vi "Trajectory Builder.vi"() -> ()   [LabVIEW 2018]
uses:
  2019 robot/Support Code/Availible Command systems for auto.ctl
  <vilib>/event_ctls.llb/lveventtype.ctl
panel:
  out "folder names":cluster{"name":string, "name":string}
  in  "Directory":bool
  in  "Tab Control":T1(tab)
  out "Duration (s)":dbl format="%#.4g"
  out "Distance (ft)":dbl format="%#.1g"
  out "WayPoints":cluster{"x":dbl, "y":dbl, "th":dbl}[](array[cluster]) {"th" format="%#_4g"}
  in  "Center Flip":bool
  in  "Snap to foot":bool
  in  "Angle Limiter":enum16{"90", "45", "15", "1"}(ring)=enum."15"
  in  "Snap robot to baseline":bool
  in  "Angular Accelerations":T2 {"Angular \nAccelerations" step=5.0}
  in  "Limits":T3={"Velocity (fps)"=6.0, "Accel (fps^2)"=15.0, "Jerk (fps^3)"=15.0} {"Jerk (fps^3)" min=0.0 step=1.0; "Accel (fps^2)" min=0.0; "Velocity (fps)" min=0.0}
  in  "Conditions":T4 {"vFinal (fps)" min=0.0; "vInitial (fps)" min=0.0}
  in  "Sample Period (s)":dbl=0.02
  in  "Unjank":bool
  in  "Turn \nAcceleration":bool=TRUE
  in  "Turn \nDeceleration":bool=TRUE
  out "Command Info":string
  in  "Reorder":bool
  in  "Commands":T5(array[cluster]) {"System" items=["Elevator", "Carriage Intake STOP", "Carriage Intake RUN"]}
  in  "Time (s)":dbl(slide) scale=-1.0..5.140000000000001 scale format="%#.1g"
  in  "Play":bool
  in  "Sub Dir 2":u16(ring)
  in  "Sub Dir 1":u16(ring) items=["Experimental", "Left", "Other", "Right"]
  out "fps":dbl[](graph)
  in  "Append":bool
  in  "Open":i32(listbox)
  in  "Filename":string
  in  "Save":bool
  in  "New":bool
  out "Picture":picture
  # "Directions:\nUse mouse to ...\n    move robot position (rectangle with arrow)\n    rotate robot (red arrow)\n    move waypoints (numbered circles)\nClick in open space to add a waypoint\nShift click to delete a waypoint\nHover over a waypoint and use arrow keys to nudge\n\nTime slider and Play button will run robot along path\nto test for collisions\n\nDirection and Destionation are folder selectors for files\n\nNew creates a new path at default location\n\nAppend creates a path"
  # "Nicotine"
  # "(20ms)"
  # "Interaction Options"
  # "Path Info"
  # "1"
  # "2"
  # "3"
  # "4"
  # "5"
  # "6"
  # "7"
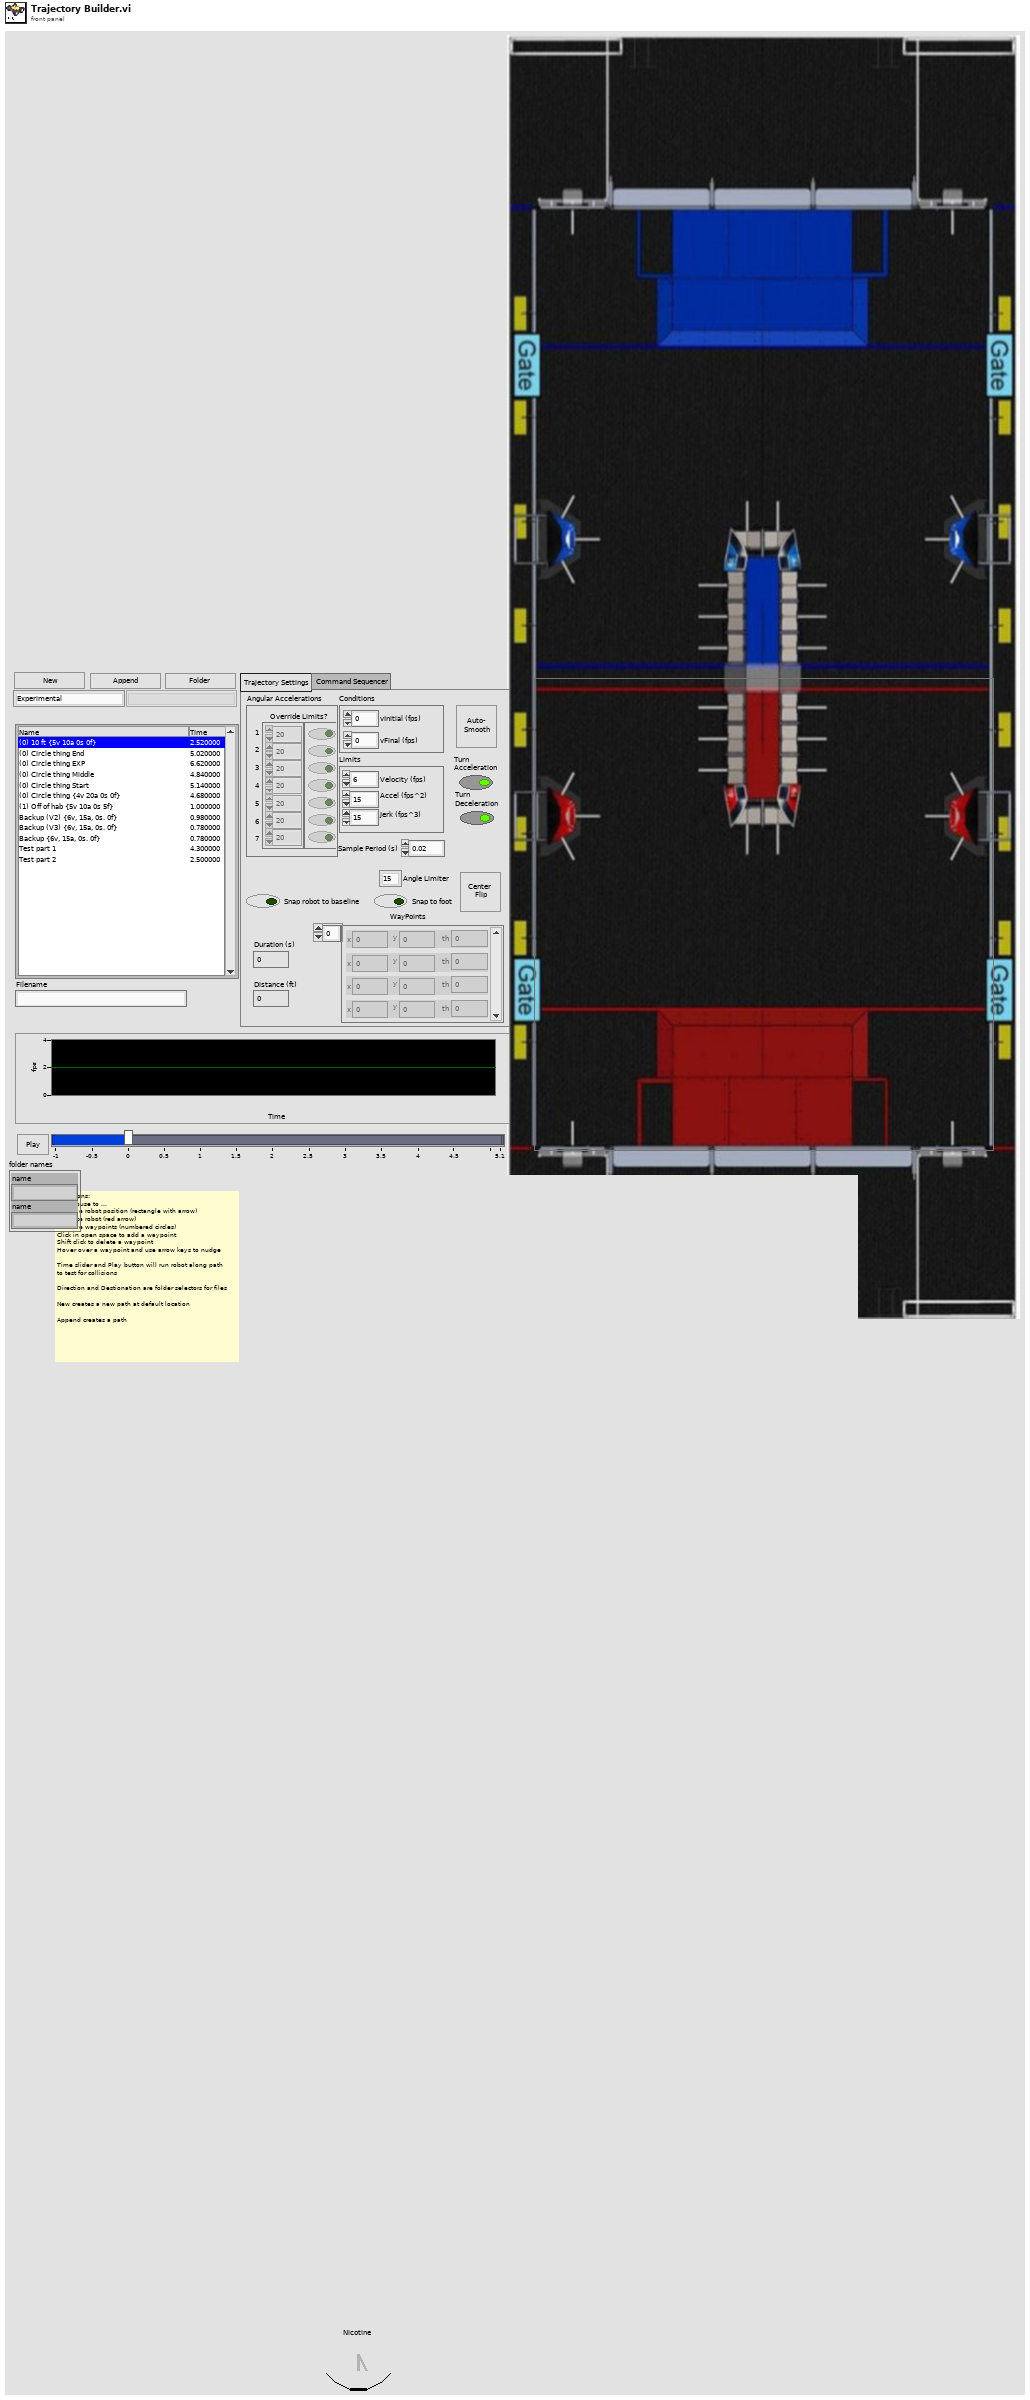
[diagram p1: front panel]
types:
  T1 = enum32{"Trajectory Settings", "Command Sequencer"}
  T2 = cluster{"Angular \nAccelerations":dbl[], "Override Limits?":bool[]}
  T3 = cluster{"Velocity (fps)":dbl, "Accel (fps^2)":dbl, "Jerk (fps^3)":dbl}
  T4 = cluster{"vInitial (fps)":dbl, "vFinal (fps)":dbl}
  T5 = cluster{"Time into Path":dbl, "System":u16, "Item Selected?":bool, "System Selection":u16}[]
  T6 = cluster{"Sample Period (s)":dbl, "Limits":cluster{"Velocity (fps)":dbl, "Acceleration (fps^2)":dbl, "Jerk (fps^3)":dbl}, "Conditions":cluster{"vInitial (fps)":dbl, "vFinal (fps)":dbl}, "output cluster":cluster{"Angular \nAccelerations":dbl[], "Override Limits?":bool[]}}
  T7 = cluster{"Segment Name":string, "Type":enum16{"Accel Straight", "Const Straight", "Blend", "Circle"}, "Traj Pos Points":cluster{"x":dbl, "y":dbl, "th":dbl}[], "Traj Vel Points":cluster{"V":dbl, "th":dbl}[], "Accel Index":i32, "Decel Index":i32}[]
  T8 = cluster{"Index":i32, "Pt Test Results":enum16{"Miss", "Rect Hit", "Arrow Hit"}}
  T9 = cluster{"Drag Object":cluster{"Index":i32, "x":dbl, "y":dbl}, "Hover Object":cluster{"Index":i32, "Pt Test Results":enum16{"Miss", "Rect Hit", "Arrow Hit"}}}
  T10 = cluster{"Trajectory Data":cluster{"Segment Name":string, "Type":enum16{"Accel Straight", "Const Straight", "Blend", "Circle"}, "Traj Pos Points":cluster{"x":dbl, "y":dbl, "th":dbl}[], "Traj Vel Points":cluster{"V":dbl, "th":dbl}[], "Accel Index":i32, "Decel Index":i32}[], "Points":cluster{"x":dbl, "y":dbl, "th":dbl}[], "Cluster":cluster{"Sample Period (s)":dbl, "Limits":cluster{"Velocity (fps)":dbl, "Acceleration (fps^2)":dbl, "Jerk (fps^3)":dbl}, "Conditions":cluster{"vInitial (fps)":dbl, "vFinal (fps)":dbl}, "output cluster":cluster{"Angular \nAccelerations":dbl[], "Override Limits?":bool[]}}}
  T11 = cluster{"Velocity":dbl, "Sample Time":dbl, "Accel":dbl}
  T12 = cluster{"Sample Period (s)":dbl, "Limits":cluster{"Velocity (fps)":dbl, "Acceleration (fps^2)":dbl, "Jerk (fps^3)":dbl}, "Conditions":cluster{"vInitial (fps)":dbl, "vFinal (fps)":dbl}}
  T13 = cluster{"Sample Period (s)":dbl, "Limits":cluster{"Velocity (fps)":dbl, "Acceleration (fps^2)":dbl, "Jerk (fps^3)":dbl}, "Conditions":cluster{"vInitial (fps)":dbl, "vFinal (fps)":dbl}, "Min Rads":dbl[]}
  T14 = typedef "Availible Command systems for auto.ctl" = u16
  T15 = cluster{"Time into Path":dbl, "System":T14, "Item Selected?":bool, "System Selection":T14}[]
  T16 = typedef "lveventtype.ctl" = enum32{"Null", "Timeout", "Annotation Menu Selection", "Annotation Menu Selection?", "App Instance Close", "App Instance Close?", "Autoscale Range Change", "Bookmark Info Change", "Cell Edit", "Cell Edit?", "Cursor Grab", "Cursor Grab?", "Cursor Menu Selection", "Cursor Menu Selection?", "Cursor Move", "Cursor Release", "Data Change", "Direction Change", "Display State Change", "Drag Ended", "Drag Enter", "Drag Leave", "Drag Over", "Drag Source Update", "Drag Starting", "Drag Starting?", "Drop", "Exec State Change", "Key Down", "Key Down?", "Key Repeat", "Key Repeat?", "Key Up", "Listbox Double Click", "Menu Activation?", "Menu Selection (App)", "Menu Selection? (App)", "Menu Selection (User)", "Mouse Down", "Mouse Down?", "Mouse Enter", "Mouse Leave", "Mouse Move", "Mouse Up", "Mouse Wheel", "NI Security User Change (App)", "Pane Size", "Panel Close", "Panel Close?", "Panel Resize", "Plot Attribute Change", "Scale Range Change", "Shortcut Menu Activation?", "Shortcut Menu Selection (App)", "Shortcut Menu Selection? (App)", "Shortcut Menu Selection (User)", "Tree Double Click", "Tree Drag", "Tree Drag?", "Tree Drop", "Tree Drop?", "Tree Item Close", "Tree Item Close?", "Tree Item Open", "Tree Item Open?", "User Event", "Value Change"}
  T17 = cluster{"Sample Period (s)":dbl, "Limits":cluster{"Velocity (fps)":dbl, "Accel (fps^2)":dbl, "Jerk (fps^3)":dbl}, "Conditions":cluster{"vInitial (fps)":dbl, "vFinal (fps)":dbl}, "Angular Accelerations":cluster{"Angular \nAccelerations":dbl[], "Override Limits?":bool[]}}
  T18 = typedef "LVPoint32TypeDef.ctl" = cluster{"Horizontal":i32, "Vertical":i32}
  T19 = cluster{"Shift":bool, "Ctrl":bool, "Alt":bool, "Cmd":bool, "Opt":bool}
  T20 = typedef "LVPositionTypeDef.ctl" = cluster{"Left":i32, "Top":i32}
  T21 = typedef "LVBoundsTypeDef.ctl" = cluster{"Width":u32, "Height":u32}
  T22 = cluster{"Velocity":dbl, "Accel":dbl, "Accel":dbl}
  T23 = cluster{"Velocity (fps)":dbl, "Acceleration (fps^2)":dbl, "Jerk (fps^3)":dbl}
  T24 = cluster{"Trajectory Data":cluster{"Segment Name":string, "Type":enum16{"Accel Straight", "Const Straight", "Blend", "Circle"}, "Traj Pos Points":cluster{"x":dbl, "y":dbl, "th":dbl}[], "Traj Vel Points":cluster{"V":dbl, "th":dbl}[], "Accel Index":i32, "Decel Index":i32}[], "Points":cluster{"x":dbl, "y":dbl, "th":dbl}[], cluster{"Sample Period (s)":dbl, "Limits":cluster{"Velocity (fps)":dbl, "Accel (fps^2)":dbl, "Jerk (fps^3)":dbl}, "Conditions":cluster{"vInitial (fps)":dbl, "vFinal (fps)":dbl}, "Angular Accelerations":cluster{"Angular \nAccelerations":dbl[], "Override Limits?":bool[]}}}
  T25 = cluster{"Snap robot to baseline":bool, "Snap to foot":bool, "Angle Limiter":enum16{"90", "45", "15", "1"}}
  T26 = cluster{i32, "Pt Test Results":enum16{"Miss", "Rect Hit", "Arrow Hit"}}
  T27 = cluster{"Drag Object":cluster{"Index":i32, "x":dbl, "y":dbl}, "Results":cluster{"Index":i32, "Pt Test Results":enum16{"Miss", "Rect Hit", "Arrow Hit"}}}
  T28 = cluster{"Trajectory Data":cluster{"Segment Name":string, "Type":enum16{"Accel Straight", "Const Straight", "Blend", "Circle"}, "Traj Pos Points":cluster{"x":dbl, "y":dbl, "th":dbl}[], "Traj Vel Points":cluster{"V":dbl, "th":dbl}[], "Accel Index":i32, "Decel Index":i32}[], "Updated Waypoints":cluster{"x":dbl, "y":dbl, "th":dbl}[], "Cluster":cluster{"Sample Period (s)":dbl, "Limits":cluster{"Velocity (fps)":dbl, "Accel (fps^2)":dbl, "Jerk (fps^3)":dbl}, "Conditions":cluster{"vInitial (fps)":dbl, "vFinal (fps)":dbl}, "Angular Accelerations":cluster{"Angular \nAccelerations":dbl[], "Override Limits?":bool[]}}}
  T29 = typedef "eventvkey.ctl" = enum16{"ASCII", "Enter", "Return", "Shift", "Ctrl", "Alt", "Cmd", "Opt", "Caps", "NumLock", "Clear", "Break", "Up", "Down", "Left", "Right", "Insert", "Delete", "Home", "End", "PageUp", "PageDown", "Escape", "Help", "Pause", "ScrollLock", "F1", "F2", "F3", "F4", "F5", "F6", "F7", "F8", "F9", "F10", "F11", "F12", "F13", "F14", "F15", "F16", "F17", "F18", "F19", "F20", "F21", "F22", "F23", "F24", "Play", "VolumeUp", "VolumeDown", "Mute", "Two Byte Char"}
  T30 = cluster{"Trajectory Data":cluster{"Segment Name":string, "Type":enum16{"Accel Straight", "Const Straight", "Blend", "Circle"}, "Traj Pos Points":cluster{"x":dbl, "y":dbl, "th":dbl}[], "Traj Vel Points":cluster{"V":dbl, "th":dbl}[], "Accel Index":i32, "Decel Index":i32}[], "Updated Waypoints":cluster{"x":dbl, "y":dbl, "th":dbl}[], cluster{"Sample Period (s)":dbl, "Limits":cluster{"Velocity (fps)":dbl, "Accel (fps^2)":dbl, "Jerk (fps^3)":dbl}, "Conditions":cluster{"vInitial (fps)":dbl, "vFinal (fps)":dbl}, "Angular Accelerations":cluster{"Angular \nAccelerations":dbl[], "Override Limits?":bool[]}}}
  T31 = cluster{"Horizontal":dbl, "Vertical":dbl, "th":dbl}
  T32 = cluster{"Name":string, "Color":u32, "Style":i32, "Point Style":i32, "Name Visible":bool, "Allow Drag":bool, "Annotation Mode":i32, "Plot":i32, "Index":i32, "Position":cluster{"X":dbl, "Y":dbl}, "X Scale":i32, "Y Scale":u32, "Show Arrow":bool, "Lock Name":bool, "Plot Area":i32, "Label Offset":cluster{"X":dbl, "Y":dbl}}[]
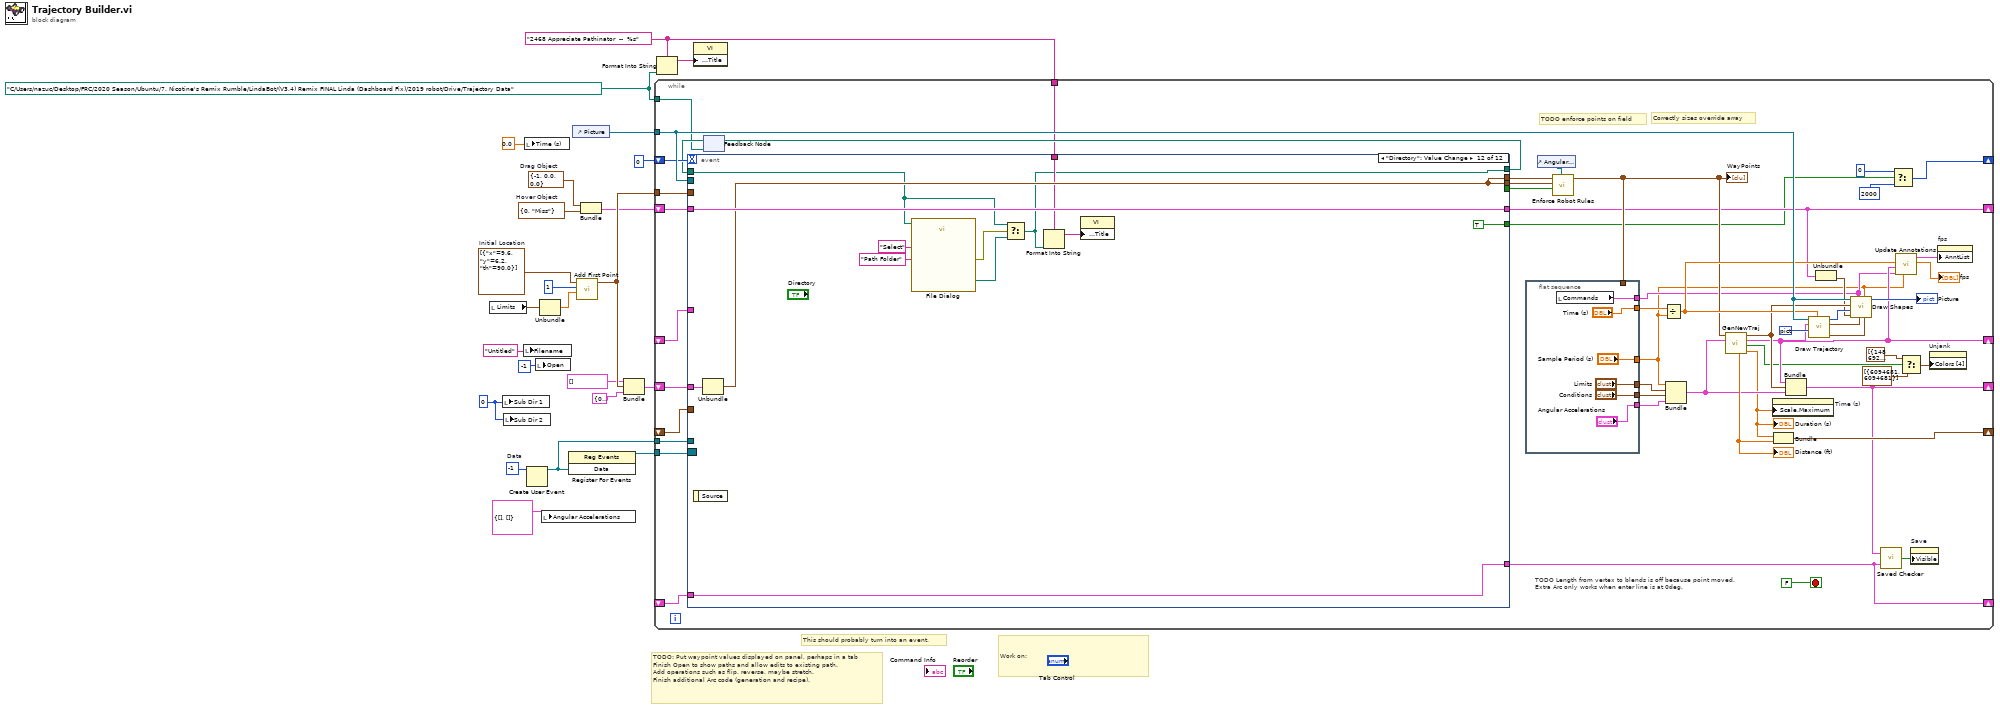
[diagram p0: block diagram]
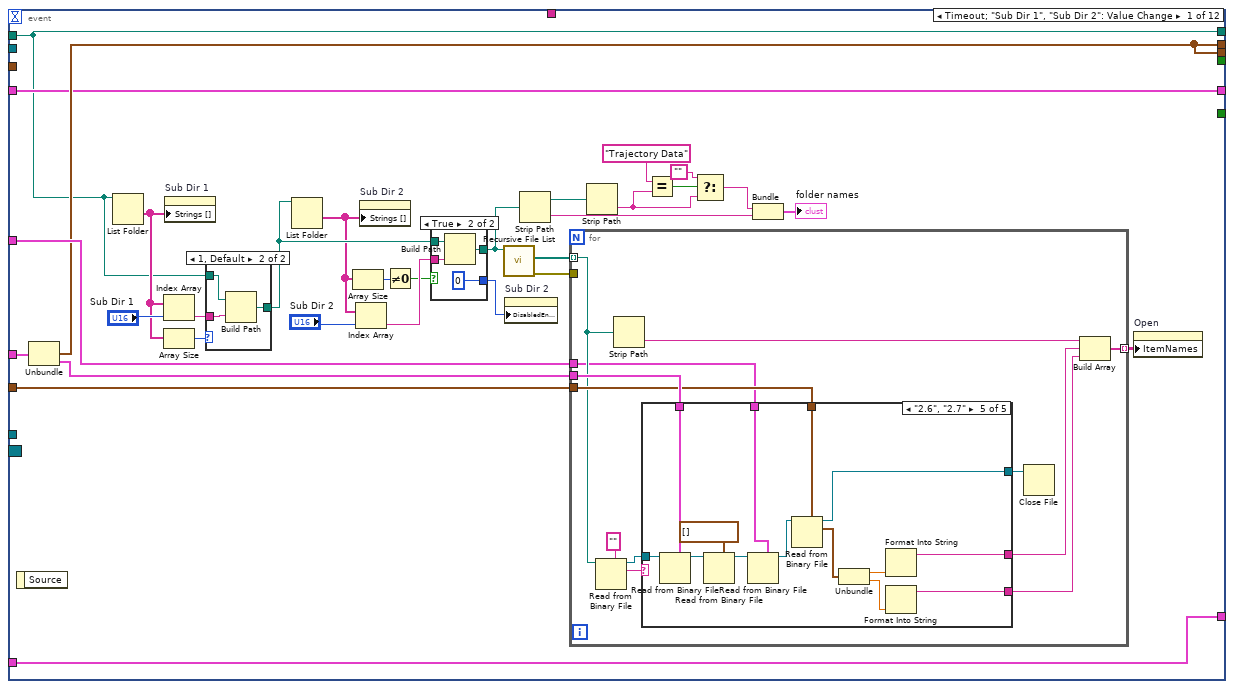
[diagram p2: hidden frame]
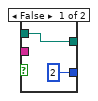
[diagram p4: hidden frame]
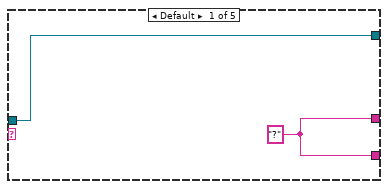
[diagram p5: hidden frame]
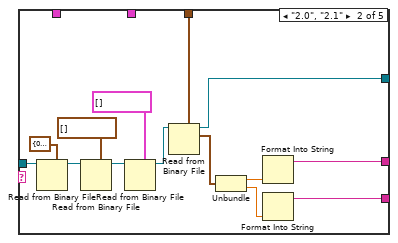
[diagram p6: hidden frame]
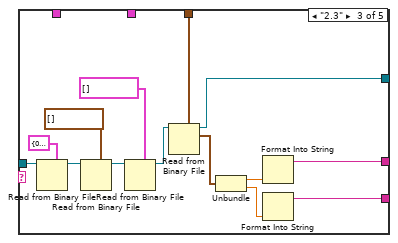
[diagram p7: hidden frame]
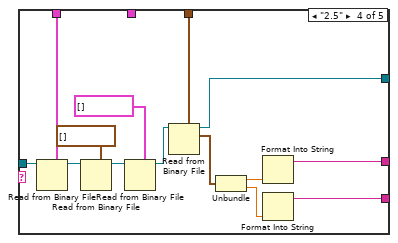
[diagram p8: hidden frame]
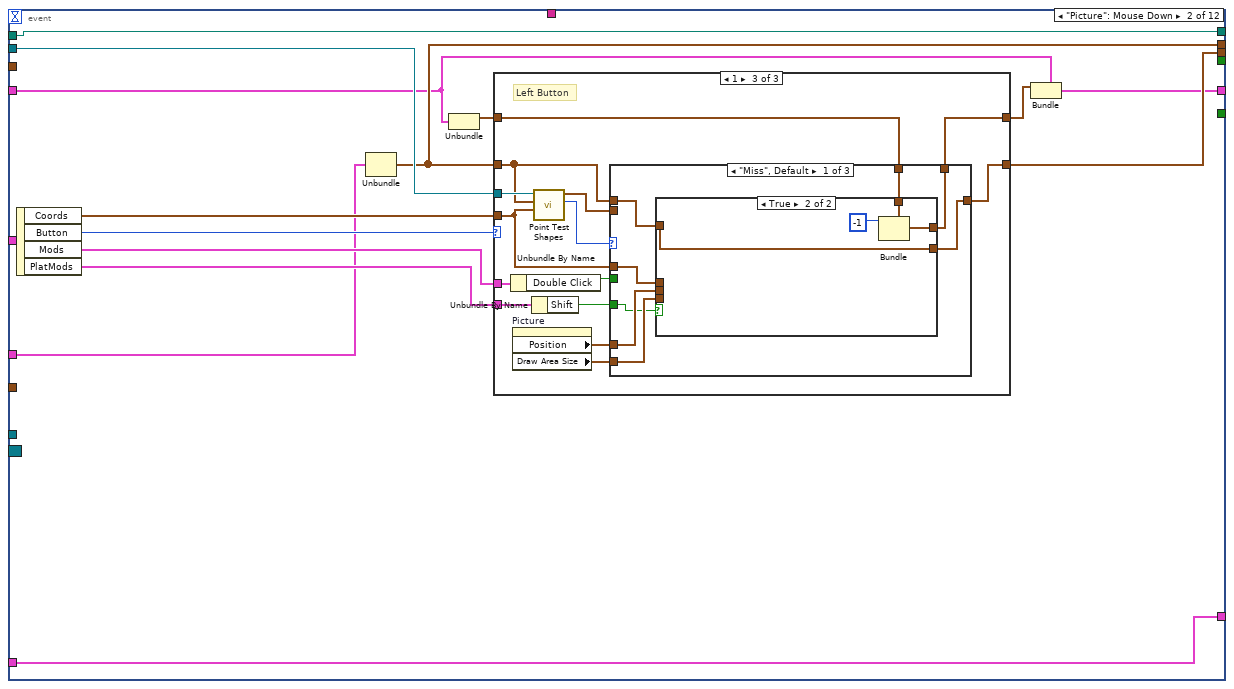
[diagram p9: hidden frame]
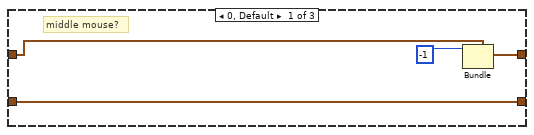
[diagram p10: hidden frame]
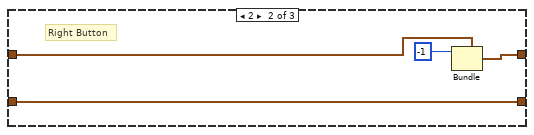
[diagram p11: hidden frame]
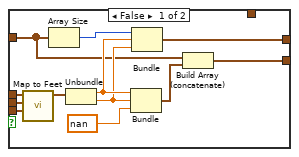
[diagram p12: hidden frame]
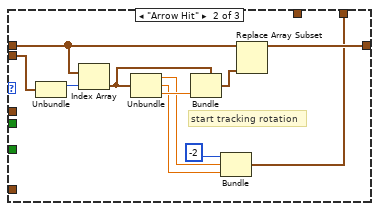
[diagram p13: hidden frame]
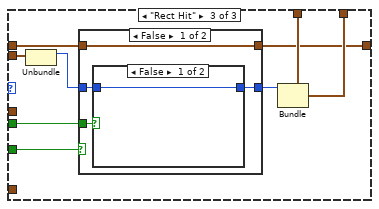
[diagram p14: hidden frame]
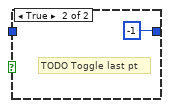
[diagram p15: hidden frame]
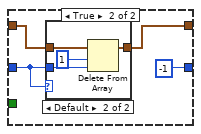
[diagram p16: hidden frame]
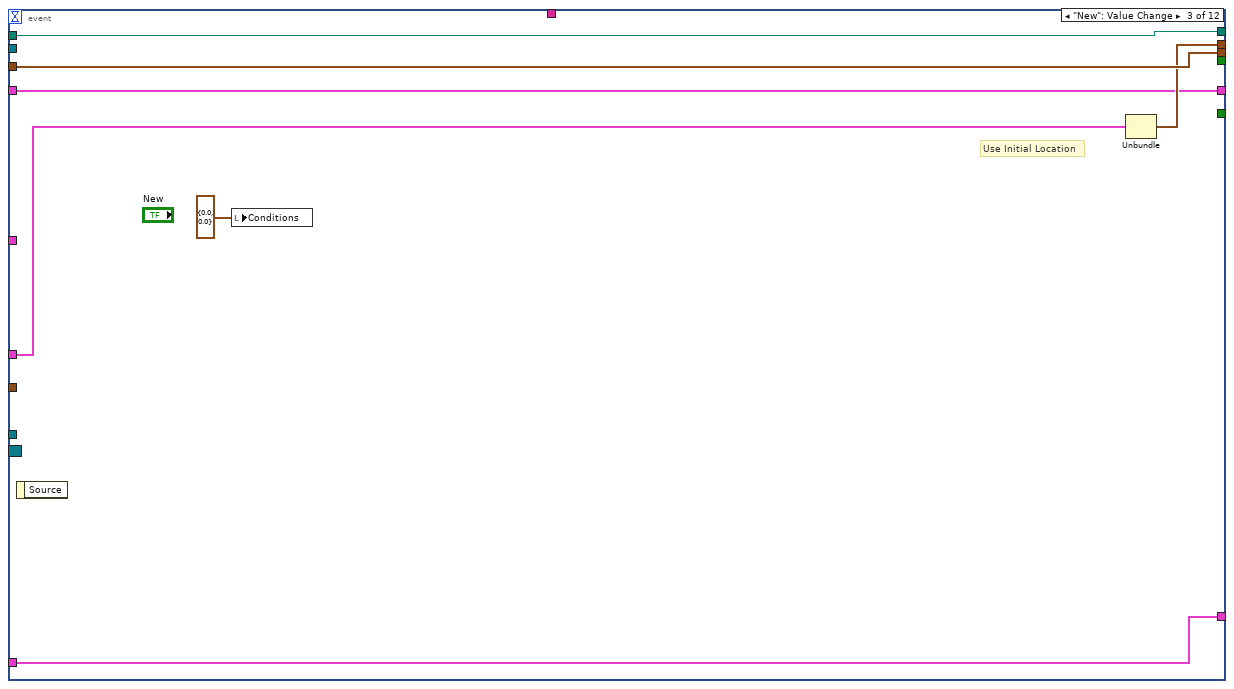
[diagram p18: hidden frame]
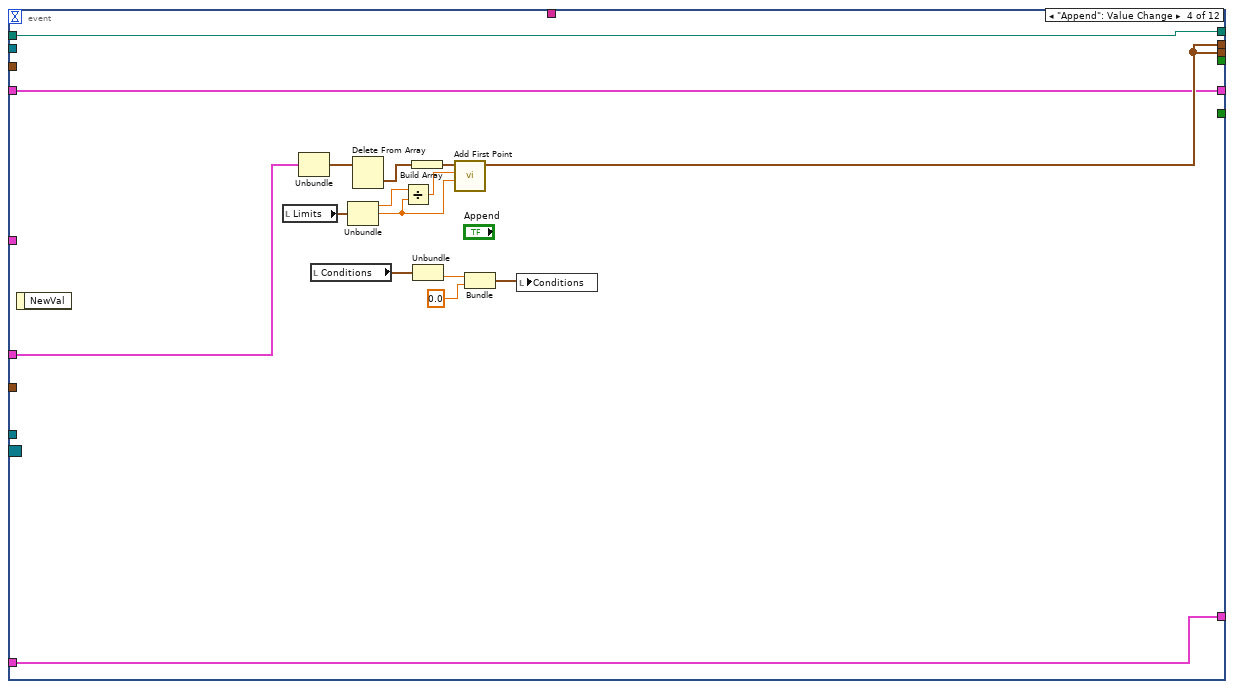
[diagram p19: hidden frame]
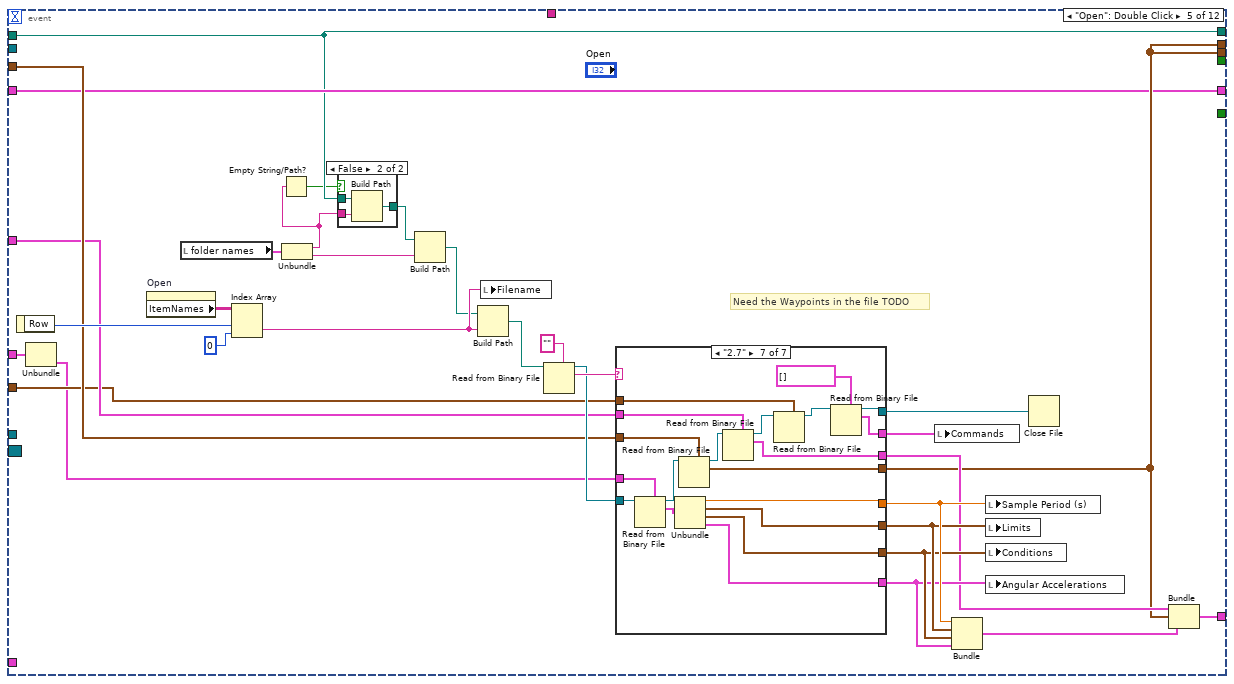
[diagram p20: hidden frame]
diagram:
  w1 = 0 ("th")
  w2 = path "C:/Users/nazuc/Desktop/FRC/2020 Season/Ubuntu/7. Nicotine's Remix Rumble/LindaBot/(V3.4) Remix FINAL Linda (Dashboard Fix)/2019 robot/Drive/Trajectory Data" ("Robot File")
  w3 = "2468 Appreciate Pathinator  --  %s" ("format string")
  w13 = -1  # Data
  w7 = T8 {"Index"=0, "Pt Test Results"=enum."Miss"}  # Hover Object
  w6 = cluster{"Index":i32, "x":dbl, "y":dbl} {"Index"=-1, "x"=0.0, "y"=0.0}  # Drag Object
  w22 = cluster{"x":dbl, "y":dbl, "th":dbl}[] [{"x"=9.6, "y"=6.2, "th"=90.0}]  # Initial Location
  # "This should probably turn into an event."
  # "Work on:"
  # "TODO: Put waypoint values displayed on panel, perhaps in a tab\nFinish Open to show paths and allow edits to existing path.\nAdd operations such as flip, reverse, maybe stretch.\nFinish additional Arc code (generation and recipe)."
  n1 = local read "Limits"() -> (w19:T3)
  n2 = local write "Sub Dir 1"(w1) -> ()
  n3 = local write "Sub Dir 2"(w1) -> ()
  n4 = local write "Filename"("Untitled" ("Filename")) -> ()
  n5 = local write "Time (s)"(0.0 ("Time")) -> ()
  n6 = Create User Event(user event datatype=w13) -> (user event=w14:refnum<user-event>)  [unwired: 1 in, 1 out]
  n7 = local write "Open"(-1) -> ()
  n8 = Unbundle(w19) -> ("Accel (fps^2)"=w18:dbl)  [unwired: 2 out]
  n9 = local write "Angular Accelerations"(T2 {"Angular \nAccelerations"=[], "Override Limits?"=[]} ("Angular Accelerations")) -> ()
  n10 = register-events(w14) -> (reference out=w15:refnum<event-registration>)  [unwired: 2 in, 1 out]
  n11 = control-ref of="Picture"() -> (w24:refnum<vi>)
  n12 = call "Add First Point.vi"("Accel (f/s^2)"=w18, "Time (s)"=1 ("th"), "Initial Points"=w22) -> ("Points"=w11:cluster{"x":dbl, "y":dbl, "th":dbl}[])  [unwired: 8 in]
  n13 = Bundle("Drag Object"=w6, "Hover Object"=w7) -> (w5:T9)  [unwired: 1 in]
  n14 = Bundle("Trajectory Data"=T7 [], "Points"=w11, "Cluster"=T6 {"Sample Period (s)"=0.02, "Limits"={"Velocity (fps)"=11.0, "Acceleration (fps^2)"=19.0, "Jerk (fps^3)"=150.0}, "Conditions"={"vInitial (fps)"=0.0, "vFinal (fps)"=0.0}, "output cluster"={"Angular \nAccelerations"=[], "Override Limits?"=[]}}) -> (w10:T10)  [unwired: 1 in]
  n15 = while {
    tunnel: w11 -> [w76]
    tunnel: w24 -> [w75]
    shift-right: [w40] -> _
    shift-left: _ -> [w69]
    shift-right: [w33] -> _
    shift-left: 0 -> [w68]
    shift-right: [w67] -> _
    shift-left: _ -> [w66]
    tunnel: w2 -> [w46]
    tunnel: w15 -> [w59]
    tunnel: w14 -> [w58]
    shift-right: [w56] -> _
    shift-left: _ -> [w57]
    shift-right: [w45] -> _
    shift-left: w10 -> [w44]
    shift-right: [w38] -> _
    shift-left: w5 -> [w39]
    tunnel: w3 -> [w36]
    stop <- FALSE stop-if-true
    # "Correctly sizes override array"
    # "TODO Length from vertex to blends is off because point moved.\nExtra Arc only works when enter line is at 0deg."
    # "TODO enforce points on field"
    n16 = feedback #1(w46) -> (w47:path)
    n17 = event shown="[11] \"Directory\": Value Change" {
      selector: w59 -> [_ _ _ _ _ _ _ _ _ _ _ _]
      dyn-events: _ -> [_ _ _ _ _ _ _ _ _ _ _ _]
      timeout: w68 -> [_ _ _ _ _ _ _ _ _ _ _ _]
      tunnel: [w95 w205 w296 w311 w323 w471 w508 w541 w575 w596 w603 w632] -> w65
      tunnel: w76 -> [_ _ w296 _ w337 _ _ _ _ _ _ _]
      tunnel: w75 -> [_ w204 _ _ _ w472 _ _ w562 _ _ _]
      tunnel: w69 -> [w99 _ _ _ w336 _ w515 _ _ _ _ _]
      tunnel: w47 -> [w93 w202 w294 w300 w315 w465 w501 w536 w576 w601 w619 w625]
      tunnel: [w95 w199 w291 w311 w323 w462 w508 w532 w560 w596 w603 w632] -> w64
      tunnel: w66 -> [w112 _ _ _ w334 _ w520 _ _ _ _ _]
      tunnel: [_ _ _ _ _ _ _ TRUE ("Flip Over Center") _ _ _ _] -> w63
      tunnel: [w93 w202 w294 w300 w315 w465 w501 w536 w576 w601 w619 w623] -> w48
      tunnel: w58 -> [_ _ _ _ _ _ _ _ _ w600 w618 _]
      tunnel: [w105 w201 w293 w301 w326 w464 w516 w535 w563 w599 w615 w634] -> w56
      tunnel: w57 -> [w105 w201 w293 w301 _ w464 _ w535 w563 w599 w615 w634]
      tunnel: w44 -> [w97 w200 w292 w299 w322 w463 w511 w533 w561 w597 w604 w633]
      tunnel: w39 -> [w94 w196 w290 w297 w320 w458 w509 w531 w558 w595 w602 w635]
      tunnel: [w94 w198 w290 w297 w320 w459 w509 w531 w558 w595 w602 w635] -> w38
      tunnel: w36 -> [_ _ _ _ _ _ _ _ _ _ _ w629]
      tunnel: [_ _ _ _ _ _ TRUE _ _ _ _ TRUE] -> w32
      event Timeout; "Sub Dir 1", "Sub Dir 2": Value Change {
        n18 = event-data() -> ()  [unwired: 1 in, 1 out]
        n19 = Unbundle(w97) -> ("Updated Waypoints"=w95:cluster{"x":dbl, "y":dbl, "th":dbl}[], "Cluster"=w96:T17)  [unwired: 1 out]
        n20 = List Folder(path=w93) -> (folder names=w101:string[])  [unwired: 3 in, 3 out]
        n21 = Index Array(array=w101, index="Sub Dir 1") -> (element=w102:string)
        n22 = Array Size(array=w101) -> (size(s)=w98:i32)
        n23 = property on="Sub Dir 1" class="Ring (strict)"("Strings []"=w101) -> ()  [unwired: 2 in, 2 out]
        n24 = case shown="1, Default" w98 {
          tunnel: w93 -> [w115 w118]
          tunnel: [w115 w117] -> w103
          tunnel: w102 -> [_ w116]
          frame 0 {
          }
          frame 1, Default {
            n25 = Build Path(base path=w118, name or relative path=w116) -> (appended path=w117:path)
          }
        }
        n26 = List Folder(path=w103) -> (folder names=w100:string[])  [unwired: 3 in, 3 out]
        n27 = Array Size(array=w100) -> (size(s)=w104:i32)
        n28 = Index Array(array=w100, index="Sub Dir 2") -> (element=w108:string)
        n29 = property on="Sub Dir 2" class="Ring (strict)"("Strings []"=w100) -> ()  [unwired: 2 in, 2 out]
        n30 = Not Equal To 0?(x=w104) -> (x != 0?=w107:bool)
        n31 = case shown="True" w107 {
          tunnel: w103 -> [w120 w124]
          tunnel: [w120 w123] -> w92
          tunnel: w108 -> [_ w122]
          tunnel: [2 0] -> w106
          frame False {
          }
          frame True {
            n32 = Build Path(base path=w124, name or relative path=w122) -> (appended path=w123:path)
          }
        }
        n33 = call <vilib>:"Recursive File List.vi"("Folder Path"=w92) -> ("error out"=w111:errorcluster, "All Files in Dir"=w114:path[])  [unwired: 6 in, 3 out]
        n34 = property on="Sub Dir 2" class="Ring (strict)"("DisabledEnum"=w106) -> ()  [unwired: 2 in, 2 out]
        n35 = Strip Path(path=w92) -> (stripped path=w91:path, name=w89:string)
        n36 = for {
          tunnel: w114 -> [w126] mode=indexing
          tunnel: [w136] -> w113 mode=indexing
          tunnel: w96 -> [w131]
          tunnel: w112 -> [w130]
          tunnel: w111 -> [_]
          tunnel: w99 -> [w125]
          n37 = Read from Binary File(5:"", 11:w126) -> (2:w134:string, 3:w133:refnum<file>)  [unwired: 4 in, 2 out]
          n38 = Strip Path(path=w126) -> (name=w127:string)  [unwired: 1 out]
          n39 = case shown="\"2.6\", \"2.7\"" w134 {
            tunnel: [w138 w152 w166 w180 w194] -> w129
            tunnel: [w138 w151 w165 w179 w193] -> w128
            tunnel: w133 -> [w137 w150 w164 w178 w192]
            tunnel: [w137 w146 w160 w174 w188] -> w132
            tunnel: w131 -> [_ _ _ w167 w182]
            tunnel: w130 -> [_ w145 w159 w173 w187]
            tunnel: w125 -> [_ _ _ _ w181]
            frame Default {
              w138 = "?"
            }
            frame "2.0", "2.1" {
              n40 = Read from Binary File(5:T11 {"Velocity"=0.0, "Sample Time"=0.0, "Accel"=0.0}, 11:w150) -> (3:w149:refnum<file>)  [unwired: 4 in, 3 out]
              n41 = Read from Binary File(5:cluster{"x":dbl, "y":dbl, "th":dbl}[] [] ("Points"), 11:w149) -> (3:w148:refnum<file>)  [unwired: 4 in, 3 out]
              n42 = Read from Binary File(5:T7 [] ("Trajectory Data"), 11:w148) -> (3:w147:refnum<file>)  [unwired: 4 in, 3 out]
              n43 = Read from Binary File(5:w145, 11:w147) -> (2:w140:cluster{"Time (s)":dbl, "Distance (ft)":dbl}, 3:w146:refnum<file>)  [unwired: 4 in, 2 out]
              n44 = Unbundle(w140) -> ("Time (s)"=w144:dbl, "Distance (ft)"=w143:dbl)
              n45 = Format Into String(w144) -> (resulting string=w152:string)  [unwired: 3 in, 1 out]
              n46 = Format Into String(w143) -> (resulting string=w151:string)  [unwired: 3 in, 1 out]
            }
            frame "2.3" {
              n47 = Read from Binary File(5:T12 {"Sample Period (s)"=0.0, "Limits"={"Velocity (fps)"=0.0, "Acceleration (fps^2)"=0.0, "Jerk (fps^3)"=0.0}, "Conditions"={"vInitial (fps)"=0.0, "vFinal (fps)"=0.0}}, 11:w164) -> (3:w163:refnum<file>)  [unwired: 4 in, 3 out]
              n48 = Read from Binary File(5:cluster{"x":dbl, "y":dbl, "th":dbl}[] [] ("Points"), 11:w163) -> (3:w162:refnum<file>)  [unwired: 4 in, 3 out]
              n49 = Read from Binary File(5:T7 [] ("Trajectory Data"), 11:w162) -> (3:w161:refnum<file>)  [unwired: 4 in, 3 out]
              n50 = Read from Binary File(5:w159, 11:w161) -> (2:w154:cluster{"Time (s)":dbl, "Distance (ft)":dbl}, 3:w160:refnum<file>)  [unwired: 4 in, 2 out]
              n51 = Unbundle(w154) -> ("Time (s)"=w158:dbl, "Distance (ft)"=w157:dbl)
              n52 = Format Into String(w158) -> (resulting string=w166:string)  [unwired: 3 in, 1 out]
              n53 = Format Into String(w157) -> (resulting string=w165:string)  [unwired: 3 in, 1 out]
            }
            frame "2.5" {
              n54 = Read from Binary File(5:w167, 11:w178) -> (3:w177:refnum<file>)  [unwired: 4 in, 3 out]
              n55 = Read from Binary File(5:cluster{"x":dbl, "y":dbl, "th":dbl}[] [] ("Points"), 11:w177) -> (3:w176:refnum<file>)  [unwired: 4 in, 3 out]
              n56 = Read from Binary File(5:T7 [] ("Trajectory Data"), 11:w176) -> (3:w175:refnum<file>)  [unwired: 4 in, 3 out]
              n57 = Read from Binary File(5:w173, 11:w175) -> (2:w168:cluster{"Time (s)":dbl, "Distance (ft)":dbl}, 3:w174:refnum<file>)  [unwired: 4 in, 2 out]
              n58 = Unbundle(w168) -> ("Time (s)"=w172:dbl, "Distance (ft)"=w171:dbl)
              n59 = Format Into String(w172) -> (resulting string=w180:string)  [unwired: 3 in, 1 out]
              n60 = Format Into String(w171) -> (resulting string=w179:string)  [unwired: 3 in, 1 out]
            }
            frame "2.6", "2.7" {
              n61 = Read from Binary File(5:w182, 11:w192) -> (3:w191:refnum<file>)  [unwired: 4 in, 3 out]
              n62 = Read from Binary File(5:cluster{"x":dbl, "y":dbl, "th":dbl}[] [] ("Points"), 11:w191) -> (3:w190:refnum<file>)  [unwired: 4 in, 3 out]
              n63 = Read from Binary File(5:w181, 11:w190) -> (3:w189:refnum<file>)  [unwired: 4 in, 3 out]
              n64 = Read from Binary File(5:w187, 11:w189) -> (2:w183:cluster{"Time (s)":dbl, "Distance (ft)":dbl}, 3:w188:refnum<file>)  [unwired: 4 in, 2 out]
              n65 = Unbundle(w183) -> ("Time (s)"=w186:dbl, "Distance (ft)"=w185:dbl)
              n66 = Format Into String(w186) -> (resulting string=w194:string)  [unwired: 3 in, 1 out]
              n67 = Format Into String(w185) -> (resulting string=w193:string)  [unwired: 3 in, 1 out]
            }
          }
          n68 = Close File(refnum=w132) -> ()  [unwired: 1 in, 2 out]
          n69 = Build Array(w127, w129, w128) -> (w136:string[])
        }
        n70 = Strip Path(path=w91) -> (name=w85:string)  [unwired: 1 out]
        n71 = Equal?(x="Trajectory Data", y=w85) -> (x = y?=w88:bool)
        n72 = Select(t="", s=w88, f=w85) -> (s? t:f=w84:string)
        n73 = Bundle("name"=w84, "name"=w89) -> (→"folder names":cluster{"name":string, "name":string})  [unwired: 1 in]
        n74 = property on="Open" class="MCListbox (strict)"("ItemNames"=w113) -> ()  [unwired: 2 in, 2 out]
      }
      event "Picture": Mouse Down {
        n75 = event-data() -> ("Coords"=w206:T18, "Button"=w208:u16, "Mods"=w207:cluster{"Double Click":bool, "Menu Key":bool}, "PlatMods"=w203:T19)  [unwired: 1 in]
        n76 = Unbundle(w200) -> ("Updated Waypoints"=w199:cluster{"x":dbl, "y":dbl, "th":dbl}[])  [unwired: 2 out]
        n77 = Unbundle(w196) -> ("Drag Object"=w195:cluster{"Index":i32, "x":dbl, "y":dbl})  [unwired: 1 out]
        n78 = case shown="1" w208 {
          tunnel: w207 -> [_ _ w220]
          tunnel: w206 -> [_ _ w225]
          tunnel: w199 -> [w212 w216 w226]
          tunnel: [w212 w216 w230] -> w205
          tunnel: w204 -> [_ _ w227]
          tunnel: w195 -> [w210 w213 w221]
          tunnel: [w209 w215 w222] -> w197
          tunnel: w203 -> [_ _ w218]
          frame 0, Default {
            # "middle mouse?"
            n79 = Bundle(cluster=w210, "Index"=-1) -> (w209:cluster{"Index":i32, "x":dbl, "y":dbl})  [unwired: 2 in]
          }
          frame 2 {
            # "Right Button"
            n80 = Bundle(cluster=w213, "Index"=-1) -> (w215:cluster{"Index":i32, "x":dbl, "y":dbl})  [unwired: 2 in]
          }
          frame 1 {
            # "Left Button"
            n81 = Unbundle By Name(w220) -> ("Double Click"=w219:bool)
            n82 = property on="Picture" class="Pict"() -> ("Position"=w229:T20, "Draw Area Size"=w228:T21)  [unwired: 2 in, 2 out]
            n83 = Unbundle By Name(w218) -> ("Shift"=w217:bool)
            n84 = call "Point Test Shapes.vi"("Coords"=w225, "Points"=w226, "Picture in"=w227) -> ("Pt Test Results"=w224:enum16{"Miss", "Rect Hit", "Arrow Hit"}, "Results"=w223:T8)  [unwired: 7 in]
            n85 = case shown="\"Miss\", Default" w224 {
              tunnel: w219 -> [_ _ w273]
              tunnel: w226 -> [w234 w262 w267]
              tunnel: w223 -> [_ w260 w274]
              tunnel: [w237 w263 w266] -> w230
              tunnel: w225 -> [w238 _ _]
              tunnel: w229 -> [w236 _ _]
              tunnel: w228 -> [w235 _ _]
              tunnel: [w232 w255 w270] -> w222
              tunnel: w221 -> [w231 _ w271]
              tunnel: w217 -> [w233 _ w268]
              frame "Miss", Default {
                n86 = case shown="True" w233 {
                  tunnel: w238 -> [w250 _]
                  tunnel: [w247 w254] -> w237
                  tunnel: w236 -> [w246 _]
                  tunnel: w235 -> [w245 _]
                  tunnel: w234 -> [w241 w254]
                  tunnel: [w240 w253] -> w232
                  tunnel: w231 -> [_ w251]
                  frame False {
                    n87 = call "Map to Feet.vi"("Draw Area Size"=w245, "Position"=w246, "Coords (px)"=w250) -> ("Point (ft)"=w244:cluster{dbl, dbl})  [unwired: 8 in]
                    n88 = Array Size(array=w241) -> (size(s)=w239:i32)
                    n89 = Unbundle(w244) -> (w243:dbl, w242:dbl)
                    n90 = Bundle(w243, w242, nan) -> (w248:cluster{dbl, dbl, dbl})  [unwired: 1 in]
                    n91 = Bundle(w239, w243, w242) -> (w240:cluster{i32, dbl, dbl})  [unwired: 1 in]
                    n92 = Build Array (concatenate)(w241, w248) -> (w247:cluster{"x":dbl, "y":dbl, "th":dbl}[])
                  }
                  frame True {
                    n93 = Bundle(cluster=w251, "Index"=-1) -> (w253:cluster{"Index":i32, "x":dbl, "y":dbl})  [unwired: 2 in]
                  }
                }
              }
              frame "Arrow Hit" {
                # "start tracking rotation"
                n94 = Unbundle(w260) -> ("Index"=w259:i32)  [unwired: 1 out]
                n95 = Index Array(array=w262, index=w259) -> (element=w261:cluster{"x":dbl, "y":dbl, "th":dbl})
                n96 = Unbundle(w261) -> ("x"=w258:dbl, "y"=w257:dbl, "th"=w265:dbl)
                n97 = Bundle(cluster=w261, "th"=w265) -> (w264:cluster{"x":dbl, "y":dbl, "th":dbl})  [unwired: 2 in]
                n98 = Bundle(-2, "x"=w258, "y"=w257) -> (w255:cluster{i32, "x":dbl, "y":dbl})  [unwired: 1 in]
                n99 = Replace Array Subset(array=w262, new element=w264) -> (w263:cluster{"x":dbl, "y":dbl, "th":dbl}[])  [unwired: 1 in]
              }
              frame "Rect Hit" {
                n100 = Unbundle(w274) -> ("Index"=w272:i32)  [unwired: 1 out]
                n101 = case shown="False" w268 {
                  tunnel: w273 -> [w278 _]
                  tunnel: w272 -> [w277 w281]
                  tunnel: [w276 -1 ("length")] -> w269
                  tunnel: w267 -> [w275 w284]
                  tunnel: [w275 w283] -> w266
                  frame False {
                    n102 = case shown="False" w278 {
                      tunnel: w277 -> [w279 _]
                      tunnel: [w279 -1] -> w276
                      frame False {
                      }
                      frame True {
                        # "TODO Toggle last pt"
                      }
                    }
                  }
                  frame True {
                    n103 = case shown="Default" w281 {
                      tunnel: w284 -> [w285 w289]
                      tunnel: w281 -> [_ w288]
                      tunnel: [w285 w286] -> w283
                      frame 0 {
                      }
                      frame Default {
                        n104 = Delete From Array(array=w289, length=1, index=w288) -> (array with subset deleted=w286:cluster{"x":dbl, "y":dbl, "th":dbl}[])  [unwired: 1 out]
                      }
                    }
                  }
                }
                n105 = Bundle(cluster=w271, "Index"=w269) -> (w270:cluster{"Index":i32, "x":dbl, "y":dbl})  [unwired: 2 in]
              }
            }
          }
        }
        n106 = Bundle(cluster=w196, "Drag Object"=w197) -> (w198:T9)  [unwired: 1 in]
      }
      event "New": Value Change {
        # "Use Initial Location"
        n107 = event-data() -> ()  [unwired: 1 in, 1 out]
        n108 = local write "Conditions"(T4 {"vInitial (fps)"=0.0, "vFinal (fps)"=0.0} ("Conditions")) -> ()
        n109 = Unbundle(w292) -> ("Updated Waypoints"=w291:cluster{"x":dbl, "y":dbl, "th":dbl}[])  [unwired: 2 out]
      }
      event "Append": Value Change {
        n110 = event-data() -> ()  [unwired: 1 in, 1 out]
        n111 = local read "Limits"() -> (w304:T3)
        n112 = Unbundle(w299) -> ("Updated Waypoints"=w298:cluster{"x":dbl, "y":dbl, "th":dbl}[])  [unwired: 2 out]
        n113 = local read "Conditions"() -> (w308:T4)
        n114 = Unbundle(w304) -> ("Velocity (fps)"=w303:dbl, "Accel (fps^2)"=w302:dbl)  [unwired: 1 out]
        n115 = Delete From Array(array=w298) -> (deleted portion=w310:cluster{"x":dbl, "y":dbl, "th":dbl})  [unwired: 2 in, 1 out]
        n116 = Divide(x=w303, y=w302) -> (x/y=w312:dbl)
        n117 = Build Array(w310) -> (w309:cluster{"x":dbl, "y":dbl, "th":dbl}[])
        n118 = Unbundle(w308) -> ("vFinal (fps)"=w307:dbl)  [unwired: 1 out]
        n119 = call "Add First Point.vi"("Accel (f/s^2)"=w302, "Time (s)"=w312, "Initial Points"=w309) -> ("Points"=w311:cluster{"x":dbl, "y":dbl, "th":dbl}[])  [unwired: 8 in]
        n120 = Bundle("vFinal (fps)"=w307, 0.0) -> (w306:cluster{"vFinal (fps)":dbl, dbl})  [unwired: 1 in]
        n121 = local write "Conditions"(w306) -> ()
      }
      event "Open": Double Click {
        # "Need the Waypoints in the file TODO"
        n122 = event-data() -> ("Row"=w342:i32)  [unwired: 1 in]
        n123 = Unbundle(w322) -> ("Cluster"=w321:T17)  [unwired: 2 out]
        n124 = property on="Open" class="MCListbox (strict)"() -> ("ItemNames"=w343:string[][])  [unwired: 2 in, 2 out]
        n125 = local read "folder names"() -> (w319:cluster{"name":string, "name":string})
        n126 = Index Array(array=w343, index (row)=w342, index (col)=0 ("disabled index (col)")) -> (element=w332:string)
        n127 = Unbundle(w319) -> ("name"=w314:string, "name"=w317:string)
        n128 = Empty String/Path?(string/path=w314) -> (empty?=w313:bool)
        n129 = case shown="False" w313 {
          tunnel: w314 -> [_ w347]
          tunnel: [w344 w346] -> w318
          tunnel: w315 -> [w344 w345]
          frame True {
          }
          frame False {
            n130 = Build Path(base path=w345, name or relative path=w347) -> (appended path=w346:path)
          }
        }
        n131 = Build Path(base path=w318, name or relative path=w317) -> (appended path=w316:path)
        n132 = Build Path(base path=w316, name or relative path=w332) -> (appended path=w333:path)
        n133 = local write "Filename"(w332) -> ()
        n134 = Read from Binary File(5:"", 11:w333) -> (2:w339:string, 3:w338:refnum<file>)  [unwired: 4 in, 2 out]
        n135 = case shown="\"2.7\"" w339 {
          tunnel: w338 -> [w350 w367 w383 w399 w419 w436 w455]
          tunnel: w321 -> [_ _ _ _ _ w425 w445]
          tunnel: w337 -> [_ w365 w381 w397 w417 w434 w453]
          tunnel: [_ w364 w380 w396 w416 w433 w452] -> w323
          tunnel: w336 -> [_ w363 w379 w395 w415 w432 w451]
          tunnel: w334 -> [_ w361 w377 w393 w413 w430 w449]
          tunnel: [w350 w359 w375 w391 w411 w428 w440] -> w335
          tunnel: [_ w357 w374 w390 w410 w427 w447] -> w331
          tunnel: [_ w356 w373 w389 w409 w426 w446] -> w330
          tunnel: [_ _ w372 w388 w408 w424 w444] -> w329
          tunnel: [T2 {"Angular \nAccelerations"=[], "Override Limits?"=[]} ("Angular Accelerations") T2 {"Angular \nAccelerations"=[], "Override Limits?"=[]} ("Angular Accelerations") T2 {"Angular \nAccelerations"=[], "Override Limits?"=[]} ("Angular Accelerations") T2 {"Angular \nAccelerations"=[], "Override Limits?"=[]} ("Angular Accelerations") w402 w423 w443] -> w328
          tunnel: [T7 [] ("Trajectory Data") w351 w369 w385 w401 w422 w442] -> w325
          tunnel: [_ _ _ _ _ _ w439] -> w324
          frame "False", Default {
          }
          frame "2.0", "2.1" {
            n136 = Read from Binary File(5:T11 {"Velocity"=0.0, "Sample Time"=0.0, "Accel"=0.0}, 11:w367) -> (2:w368:T11, 3:w366:refnum<file>)  [unwired: 4 in, 2 out]
            n137 = Read from Binary File(5:w365, 11:w366) -> (2:w364:cluster{"x":dbl, "y":dbl, "th":dbl}[], 3:w362:refnum<file>)  [unwired: 4 in, 2 out]
            n138 = Unbundle(w368) -> ("Velocity"=w355:dbl, "Sample Time"=w357:dbl, "Accel"=w354:dbl)
            n139 = Read from Binary File(5:w363, 11:w362) -> (2:w351:T7, 3:w360:refnum<file>)  [unwired: 4 in, 2 out]
            n140 = Read from Binary File(5:w361, 11:w360) -> (3:w359:refnum<file>)  [unwired: 4 in, 3 out]
            n141 = Bundle("Velocity"=w355, "Accel"=w354, "Accel"=1000.0) -> (w356:T22)  [unwired: 1 in]
          }
          frame "2.3" {
            n142 = Read from Binary File(5:T12 {"Sample Period (s)"=0.0, "Limits"={"Velocity (fps)"=0.0, "Acceleration (fps^2)"=0.0, "Jerk (fps^3)"=0.0}, "Conditions"={"vInitial (fps)"=0.0, "vFinal (fps)"=0.0}}, 11:w383) -> (2:w384:T12, 3:w382:refnum<file>)  [unwired: 4 in, 2 out]
            n143 = Unbundle(w384) -> ("Sample Period (s)"=w374:dbl, "Limits"=w373:T23, "Conditions"=w372:T4)
            n144 = Read from Binary File(5:w381, 11:w382) -> (2:w380:cluster{"x":dbl, "y":dbl, "th":dbl}[], 3:w378:refnum<file>)  [unwired: 4 in, 2 out]
            n145 = Read from Binary File(5:w379, 11:w378) -> (2:w369:T7, 3:w376:refnum<file>)  [unwired: 4 in, 2 out]
            n146 = Read from Binary File(5:w377, 11:w376) -> (3:w375:refnum<file>)  [unwired: 4 in, 3 out]
          }
          frame "2.4" {
            n147 = Read from Binary File(5:T12 {"Sample Period (s)"=0.0, "Limits"={"Velocity (fps)"=0.0, "Acceleration (fps^2)"=0.0, "Jerk (fps^3)"=0.0}, "Conditions"={"vInitial (fps)"=0.0, "vFinal (fps)"=0.0}}, 11:w399) -> (2:w400:T12, 3:w398:refnum<file>)  [unwired: 4 in, 2 out]
            n148 = Unbundle(w400) -> ("Sample Period (s)"=w390:dbl, "Limits"=w389:T23, "Conditions"=w388:T4)
            n149 = Read from Binary File(5:w397, 11:w398) -> (2:w396:cluster{"x":dbl, "y":dbl, "th":dbl}[], 3:w394:refnum<file>)  [unwired: 4 in, 2 out]
            n150 = Read from Binary File(5:w395, 11:w394) -> (2:w385:T7, 3:w392:refnum<file>)  [unwired: 4 in, 2 out]
            n151 = Read from Binary File(5:w393, 11:w392) -> (3:w391:refnum<file>)  [unwired: 4 in, 3 out]
          }
          frame "2.5" {
            n152 = Read from Binary File(5:T13 {"Sample Period (s)"=0.0, "Limits"={"Velocity (fps)"=0.0, "Acceleration (fps^2)"=0.0, "Jerk (fps^3)"=0.0}, "Conditions"={"vInitial (fps)"=0.0, "vFinal (fps)"=0.0}, "Min Rads"=[20.0, 20.0, 20.0, 20.0, 20.0]}, 11:w419) -> (2:w420:T13, 3:w418:refnum<file>)  [unwired: 4 in, 2 out]
            n153 = Unbundle(w420) -> ("Sample Period (s)"=w410:dbl, "Limits"=w409:T23, "Conditions"=w408:T4, "Min Rads"=w404:dbl[])
            n154 = Array Size(array=w404) -> (size(s)=w405:i32)
            n155 = for {
              N: w405 -> [_]
              tunnel: [TRUE] -> w403 mode=indexing
            }
            n156 = Read from Binary File(5:w417, 11:w418) -> (2:w416:cluster{"x":dbl, "y":dbl, "th":dbl}[], 3:w414:refnum<file>)  [unwired: 4 in, 2 out]
            n157 = Read from Binary File(5:w415, 11:w414) -> (2:w401:T7, 3:w412:refnum<file>)  [unwired: 4 in, 2 out]
            n158 = Bundle(cluster=T2 {"Angular \nAccelerations"=[], "Override Limits?"=[]} ("Angular Accelerations"), "Angular \nAccelerations"=w404, "Override Limits?"=w403) -> (w402:T2)
            n159 = Read from Binary File(5:w413, 11:w412) -> (3:w411:refnum<file>)  [unwired: 4 in, 3 out]
          }
          frame "2.6" {
            n160 = Read from Binary File(5:w425, 11:w436) -> (2:w437:T17, 3:w435:refnum<file>)  [unwired: 4 in, 2 out]
            n161 = Unbundle(w437) -> ("Sample Period (s)"=w427:dbl, "Limits"=w426:T3, "Conditions"=w424:T4, "Angular Accelerations"=w423:T2)
            n162 = Read from Binary File(5:w434, 11:w435) -> (2:w433:cluster{"x":dbl, "y":dbl, "th":dbl}[], 3:w431:refnum<file>)  [unwired: 4 in, 2 out]
            n163 = Read from Binary File(5:w432, 11:w431) -> (2:w422:T7, 3:w429:refnum<file>)  [unwired: 4 in, 2 out]
            n164 = Read from Binary File(5:w430, 11:w429) -> (3:w428:refnum<file>)  [unwired: 4 in, 3 out]
          }
          frame "2.7" {
            n165 = Read from Binary File(5:w445, 11:w455) -> (2:w456:T17, 3:w454:refnum<file>)  [unwired: 4 in, 2 out]
            n166 = Unbundle(w456) -> ("Sample Period (s)"=w447:dbl, "Limits"=w446:T3, "Conditions"=w444:T4, "Angular Accelerations"=w443:T2)
            n167 = Read from Binary File(5:w453, 11:w454) -> (2:w452:cluster{"x":dbl, "y":dbl, "th":dbl}[], 3:w450:refnum<file>)  [unwired: 4 in, 2 out]
            n168 = Read from Binary File(5:w451, 11:w450) -> (2:w442:T7, 3:w448:refnum<file>)  [unwired: 4 in, 2 out]
            n169 = Read from Binary File(5:w449, 11:w448) -> (3:w441:refnum<file>)  [unwired: 4 in, 3 out]
            n170 = Read from Binary File(5:T15 [] ("Commands"), 11:w441) -> (2:w439:T15, 3:w440:refnum<file>)  [unwired: 4 in, 2 out]
          }
        }
        n171 = local write "Commands"(w324) -> ()
        n172 = Bundle("Sample Period (s)"=w331, "Limits"=w330, "Conditions"=w329, "Angular Accelerations"=w328) -> (w327:T17)  [unwired: 1 in]
        n173 = local write "Sample Period (s)"(w331) -> ()
        n174 = local write "Limits"(w330) -> ()
        n175 = local write "Conditions"(w329) -> ()
        n176 = local write "Angular Accelerations"(w328) -> ()
        n177 = Close File(refnum=w335) -> ()  [unwired: 1 in, 2 out]
        n178 = Bundle("Trajectory Data"=w325, "Points"=w323, w327) -> (w326:T24)  [unwired: 1 in]
      }
      event "Picture": Mouse Move; "Picture": Mouse Up {
        n179 = event-data() -> ("Type"=w470:T16, "Coords"=w473:T18)  [unwired: 1 in]
        n180 = Unbundle(w458) -> ("Drag Object"=w457:cluster{"Index":i32, "x":dbl, "y":dbl})  [unwired: 1 out]
        n181 = Unbundle(w463) -> ("Updated Waypoints"=w462:cluster{"x":dbl, "y":dbl, "th":dbl}[])  [unwired: 2 out]
        n182 = Unbundle(w457) -> ("Index"=w469:i32)  [unwired: 2 out]
        n183 = case shown="Default" w469 {
          selector: w469 -> [w483 _]
          tunnel: w473 -> [w492 w499]
          tunnel: w472 -> [w478 w498]
          tunnel: [w490 w497] -> w460
          tunnel: [w487 w496] -> w471
          tunnel: w462 -> [w488 w496]
          tunnel: [w484 w495] -> w461
          tunnel: w457 -> [w474 w495]
          tunnel: w470 -> [w485 _]
          tunnel: "Snap to foot" -> [w480 _]
          tunnel: "Snap robot to baseline" -> [w481 _]
          tunnel: "Angle Limiter" -> [w482 _]
          frame Default {
            # "Mouse up changes indes to break tracking,\notherwise update coords"
            n184 = property on="Picture" class="Pict"() -> ("Position"=w493:T20, "Draw Area Size"=w494:T21)  [unwired: 2 in, 2 out]
            n185 = Bundle("Snap robot to baseline"=w481, "Snap to foot"=w480, "Angle Limiter"=w482) -> (w479:T25)  [unwired: 1 in]
            n186 = call "Map to Feet.vi"("Draw Area Size"=w494, "Position"=w493, "Coords (px)"=w492) -> ("Point (ft)"=w491:cluster{dbl, dbl})  [unwired: 8 in]
            n187 = Equal?(x=lveventtype."Mouse Up" ("Type"), y=w485) -> (x = y?=w477:bool)
            n188 = call "Handle Pos and Rot.vi"("Mouse Up"=w477, "Picture in"=w478, "Option"=w479, "Coord (ft)"=w491, "Index"=w483, "Points in"=w488) -> ("Points out"=w487:cluster{"x":dbl, "y":dbl, "th":dbl}[])  [unwired: 5 in]
            n189 = Bundle(cluster=w474, "Index"=-1) -> (w475:cluster{"Index":i32, "x":dbl, "y":dbl})  [unwired: 2 in]
            n190 = Bundle(w483, "Pt Test Results"=enum16{"Miss", "Rect Hit", "Arrow Hit"}."Rect Hit") -> (w490:T26)  [unwired: 1 in]
            n191 = Select(t=w475, s=w477, f=w474) -> (s? t:f=w484:cluster{"Index":i32, "x":dbl, "y":dbl})
          }
          frame -1 {
            n192 = call "Point Test Shapes.vi"("Coords"=w499, "Points"=w496, "Picture in"=w498) -> ("Results"=w497:T8)  [unwired: 7 in, 1 out]
          }
        }
        n193 = Bundle("Drag Object"=w461, "Results"=w460) -> (w459:T27)  [unwired: 1 in]
      }
      event "Save": Value Change {
        n194 = event-data() -> ()  [unwired: 1 in, 1 out]
        n195 = Unbundle(w511) -> ("Updated Waypoints"=w508:cluster{"x":dbl, "y":dbl, "th":dbl}[], "Cluster"=w510:T17)  [unwired: 1 out]
        n196 = local read "folder names"() -> (w507:cluster{"name":string, "name":string})
        n197 = Unbundle(w507) -> ("name"=w502:string, "name"=w506:string)
        n198 = Empty String/Path?(string/path=w502) -> (empty?=w503:bool)
        n199 = case shown="False" w503 {
          tunnel: w502 -> [_ w528]
          tunnel: [w525 w527] -> w500
          tunnel: w501 -> [w525 w526]
          frame True {
          }
          frame False {
            n200 = Build Path(base path=w526, name or relative path=w528) -> (appended path=w527:path)
          }
        }
        n201 = Build Path(base path=w500, name or relative path=w506) -> (appended path=w505:path)
        n202 = Build Path(base path=w505, name or relative path="Filename") -> (appended path=w519:path)
        n203 = Write to Binary File(file (use dialog)=w519, data="2.7") -> (refnum out=w518:refnum<file>)  [unwired: 4 in, 2 out]
        n204 = Write to Binary File(file (use dialog)=w518, data=w510) -> (refnum out=w523:refnum<file>)  [unwired: 4 in, 2 out]
        n205 = Write to Binary File(file (use dialog)=w523, data=w508) -> (refnum out=w522:refnum<file>)  [unwired: 4 in, 2 out]
        n206 = Write to Binary File(file (use dialog)=w522, data=w515) -> (refnum out=w521:refnum<file>)  [unwired: 4 in, 2 out]
        n207 = Bundle("Trajectory Data"=w515, "Updated Waypoints"=w508, "Cluster"=w510) -> (w516:T28)  [unwired: 1 in]
        n208 = Write to Binary File(file (use dialog)=w521, data=w520) -> (refnum out=w514:refnum<file>)  [unwired: 4 in, 2 out]
        n209 = Write to Binary File(file (use dialog)=w514, data="Commands") -> (refnum out=w513:refnum<file>)  [unwired: 4 in, 2 out]
        n210 = Close File(refnum=w513) -> ()  [unwired: 1 in, 2 out]
      }
      event "Time (s)", "Snap to foot", "Angle Limiter", "Snap robot to baseline", "Limits", "Sample Period (s)", "Center Flip", "Conditions", "Commands", "Unjank", "Angular Accelerations": Value Change {
        # "Changes to any of these control will run the diagram to update the preview"
        n211 = event-data() -> ("CtlRef"=w539:refnum<vi>)  [unwired: 1 in]
        n212 = control-ref of="Center Flip"() -> (w540:refnum<vi>)
        n213 = Equal?(x=w540, y=w539) -> (x = y?=w538:bool)
        n214 = case shown="True" "Unjank" {
          tunnel: w533 -> [_ w545]
          tunnel: "Turn \nAcceleration" -> [_ w543]
          tunnel: "Turn \nDeceleration" -> [_ w542]
          frame False {
          }
          frame True {
            n215 = call "Turn Smother.vi"("Ignore Deceleration"=w542, "Ignore Acceleration"=w543, "input cluster"=w545) -> ("Angular Accelerations"=w544:T2)
            n216 = local write "Angular Accelerations"(w544) -> ()
          }
        }
        n217 = Unbundle(w533) -> ("Updated Waypoints"=w532:cluster{"x":dbl, "y":dbl, "th":dbl}[])  [unwired: 2 out]
        n218 = case shown="True" w538 {
          tunnel: w532 -> [w546 w548]
          tunnel: [w546 w547] -> w541
          frame False {
          }
          frame True {
            n219 = for {
              tunnel: w548 -> [w556] mode=indexing
              tunnel: [w549] -> w547 mode=indexing
              n220 = Unbundle(w556) -> ("x"=w555:dbl, "y"=w551:dbl, "th"=w550:dbl)
              n221 = Negate(x=w555) -> (-x=w554:dbl)
              n222 = Add(x=27.0 ("y"), y=w554) -> (x+y=w552:dbl)
              n223 = Bundle(w552, "y"=w551, "th"=w550) -> (w549:cluster{dbl, "y":dbl, "th":dbl})  [unwired: 1 in]
            }
          }
        }
      }
      event Key Down?; event type 5.0.x8000000b {
        n224 = event-data() -> ("VKey"=w567:T29)  [unwired: 1 in]
        n225 = local read "Snap robot to baseline"() -> (w574:bool)
        n226 = Unbundle(w561) -> ("Updated Waypoints"=w560:cluster{"x":dbl, "y":dbl, "th":dbl}[])  [unwired: 2 out]
        n227 = local read "Angle Limiter"() -> (w572:enum16{"90", "45", "15", "1"})
        n228 = local read "Snap to foot"() -> (w573:bool)
        n229 = Unbundle(w558) -> ("Hover Object"=w559:T8)  [unwired: 1 out]
        n230 = case shown="\"Down\"" w567 {
          tunnel: [cluster{dbl, dbl} {0.0, 0.0} ("Coord (ft)") cluster{dbl, dbl} {0.0, 0.1} ("Coord (ft)") cluster{dbl, dbl} {0.0, -0.1} ("Coord (ft)") cluster{dbl, dbl} {-0.1, 0.0} ("Coord (ft)") cluster{dbl, dbl} {0.1, 0.0} ("Coord (ft)")] -> w569
          tunnel: [_ w587 w589 w591 w593] -> w565
          tunnel: TRUE ("Delta") -> [_ w587 w589 w591 w593]
          frame Default {
          }
          frame "Up" {
          }
          frame "Down" {
          }
          frame "Left" {
          }
          frame "Right" {
          }
        }
        n231 = Unbundle(w559) -> ("Index"=w557:i32, "Pt Test Results"=w566:enum16{"Miss", "Rect Hit", "Arrow Hit"})
        n232 = Bundle("Snap robot to baseline"=w574, "Snap to foot"=w573, "Angle Limiter"=w572) -> (w571:T25)  [unwired: 1 in]
        n233 = case shown="\"Rect Hit\", Default" w566 {
          tunnel: [w577 w585] -> w575
          tunnel: w562 -> [_ w584]
          tunnel: w571 -> [_ w583]
          tunnel: w560 -> [w577 w582]
          tunnel: TRUE ("Delta") -> [_ w581]
          tunnel: w569 -> [_ w580]
          tunnel: w565 -> [_ w579]
          tunnel: [_ w579] -> w564
          tunnel: w557 -> [_ w578]
          frame "Miss" {
          }
          frame "Rect Hit", Default {
            n234 = call "Handle Pos and Rot.vi"("Delta"=w581, "Picture in"=w584, "Option"=w583, "Coord (ft)"=w580, "Index"=w578, "Points in"=w582) -> ("Points out"=w585:cluster{"x":dbl, "y":dbl, "th":dbl}[])  [unwired: 5 in]
          }
        }
        n235 = event-data("Discard?"=w564) -> ()  [unwired: 1 in, 1 out]
      }
      event "Play": Value Change {
        n236 = event-data() -> ()  [unwired: 1 in, 1 out]
        n237 = Unbundle(w597) -> ("Updated Waypoints"=w596:cluster{"x":dbl, "y":dbl, "th":dbl}[])  [unwired: 2 out]
        n238 = Tick Count (ms)() -> (millisecond timer value=w598:u32)
        n239 = Generate User Event(user event=w600, event data cluster=w598) -> ()  [unwired: 2 in, 2 out]
      }
      event User Event {
        n240 = event-data() -> ("Data"=w611:i32)  [unwired: 1 in]
        n241 = Unbundle(w604) -> ("Updated Waypoints"=w603:cluster{"x":dbl, "y":dbl, "th":dbl}[])  [unwired: 2 out]
        n242 = Tick Count (ms)() -> (millisecond timer value=w614:u32)
        n243 = Subtract(x=w614, y=w611) -> (x-y=w613:u32)
        n244 = Multiply(x=w613, y=0.001) -> (x*y=w610:dbl)
        n245 = local read "Duration (s)"() -> (w616:dbl)
        n246 = Quotient & Remainder(x=w610, y=0.02) -> (floor(x/y)=w608:dbl)  [unwired: 1 out]
        n247 = Multiply(x=0.02, y=w608) -> (x*y=w607:dbl)
        n248 = Less Or Equal?(x=w607, y=w616) -> (x <= y?=w617:bool)
        n249 = case shown="True" w617 {
          tunnel: w618 -> [_ w622]
          tunnel: w611 -> [_ w620]
          tunnel: w607 -> [_ w621]
          frame False {
          }
          frame True {
            n250 = local write "Time (s)"(w621) -> ()
            n251 = Generate User Event(user event=w622, event data cluster=w620) -> ()  [unwired: 2 in, 2 out]
          }
        }
        n252 = Wait (ms)(milliseconds to wait=u32 50) -> ()  [unwired: 1 out]
      }
      event "Directory": Value Change {
        n253 = event-data() -> ()  [unwired: 1 in, 1 out]
        n254 = Unbundle(w633) -> ("Updated Waypoints"=w632:cluster{"x":dbl, "y":dbl, "th":dbl}[])  [unwired: 2 out]
        n255 = call "File Dialog"("start path"=w625, "prompt"="Path Folder", "button label"="Select") -> ("selected path"=w624:path, "error out"=w626:errorcluster)  [unwired: 9 in, 2 out]
        n256 = Select(t=w625, s=w626, f=w624) -> (s? t:f=w623:path)
        n257 = Format Into String(format string=w629, w623) -> (resulting string=w630:string)  [unwired: 2 in, 1 out]
        n258 = property class="VI"("Front Panel.Title"=w630) -> ()  [unwired: 2 in, 2 out]
      }
    }
    n259 = feedback-in #1(w48) -> ()
    n260 = flat-sequence {
      tunnel: ["Time (s)"] -> w72
      tunnel: ["Sample Period (s)"] -> w25
      tunnel: ["Limits"] -> w54
      tunnel: ["Conditions"] -> w51
      tunnel: [w79] -> w26
      tunnel: ["Angular Accelerations"] -> w43
      tunnel: w42 -> [_]
      frame #0 {
        n261 = local read "Commands"() -> (w79:T5)
      }
    }
    n262 = control-ref of="Angular Accelerations"() -> (w41:refnum<vi>)
    n263 = call "Enforce Robot Rules.vi"("Clust Refnum"=w41, "Disable"=w63, "New Points"=w65, "Original Points"=w64) -> ("Points out"=w42:cluster{"x":dbl, "y":dbl, "th":dbl}[])  [unwired: 7 in]
    "WayPoints" <- w42
    n264 = Divide(x=w72, y=w25) -> (x/y=w61:dbl)
    n265 = Bundle("Sample Period (s)"=w25, "Limits"=w54, "Conditions"=w51, "Angular Accelerations"=w43) -> (w50:T17)  [unwired: 1 in]
    n266 = call "GenNewTraj.vi"("Parameters"=w50, "Points in"=w42) -> ("Time (s)"=w49:dbl, "Valid"=w27:bool, "Trajectory Data"=w40:T7, "Updated Waypoints"=w52:cluster{"x":dbl, "y":dbl, "th":dbl}[], "Distance (ft)"=w53:dbl)  [unwired: 5 in]
    "Duration (s)" <- w49
    "Distance (ft)" <- w53
    n267 = property on="Time (s)" class="Slide (strict)"("Scale.Maximum"=w49) -> ()  [unwired: 2 in, 2 out]
    n268 = Bundle("Time (s)"=w49, "Distance (ft)"=w53) -> (w67:cluster{"Time (s)":dbl, "Distance (ft)":dbl})  [unwired: 1 in]
    n269 = Bundle("Trajectory Data"=w40, "Updated Waypoints"=w52, w50) -> (w45:T30)  [unwired: 1 in]
    n270 = call "Draw Trajectory.vi"("Robot Index"=w61, "new picture in"=picture data[5B] ("new picture"), "Trajectory Data"=w40, "Picture in"=w75) -> ("Path Points"=w55:cluster{"x":dbl, "y":dbl}[], "Output Point"=w71:T31, "new picture"=w73:picture)  [unwired: 5 in]
    n271 = Unbundle(w38) -> ("Hover Object"=w37:T8)  [unwired: 1 out]
    n272 = call "Draw Shapes.vi"("Path Points"=w55, "Sample Period (s)"=w25, "Output Point"=w71, "Commands"=w26, "Results"=w37, "new picture in"=w73, "Points"=w52, "Picture in"=w75) -> ("new picture out"=→"Picture":picture)  [unwired: 3 in]
    n273 = call "Saved Checker.vi"("comp A"=w56, "comp B"=w45) -> ("Unsaved"=w31:bool)
    n274 = Select(t=0, s=w32, f=2000) -> (s? t:f=w33:i32)
    n275 = call "Update Annotations.vi"("Sample Period"=w25, "Commands"=w26, "Trajectory Data"=w40, "Robot Pt Index"=w61) -> ("Velocity Trace"=→"fps":dbl[], "Annotation Data"=w60:T32)  [unwired: 6 in]
    n276 = Select(t=cluster{u32, u32}[] [{14869218, 14869218}] ("Colors [4]"), s=w27, f=cluster{u32, u32}[] [{6094681, 6094681}] ("Colors [4]")) -> (s? t:f=w30:cluster{u32, u32}[])
    n277 = property on="Save" class="Bool"("Visible"=w31) -> ()  [unwired: 2 in, 2 out]
    n278 = property on="Unjank" class="Bool"("Colors [4]"=w30) -> ()  [unwired: 2 in, 2 out]
    n279 = property on="fps" class="WFGraph (strict)"("AnntList"=w60) -> ()  [unwired: 2 in, 2 out]
  }
  n280 = Format Into String(format string=w3, w2) -> (resulting string=w4:string)  [unwired: 2 in, 1 out]
  n281 = property class="VI"("Front Panel.Title"=w4) -> ()  [unwired: 2 in, 2 out]
